vi "channel.data_type.vi"(8 "error in":errorcluster, 11 "Channel in":refnum<class "Channel.lvclass">) -> (0 "error out":errorcluster, 2 "type":i32, 3 "Channel out":refnum<class "Channel.lvclass">)   [LabVIEW 2020, in "Channel.lvclass"]
doc: "Returns the channel's data type."
uses:
  Channel.lvclass
  Channel.lvclass/Channel.ctl
  client.lvlib
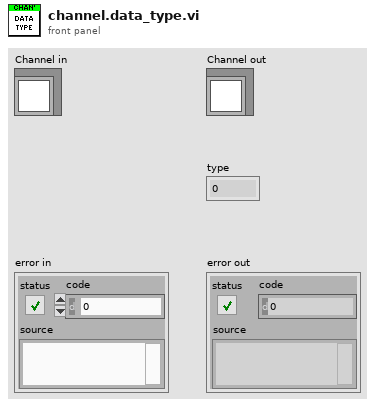
[diagram p1: front panel]
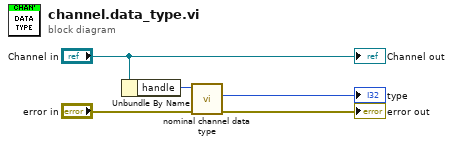
[diagram p0: block diagram]
diagram:
  n1 = Unbundle By Name("Channel in") -> ("handle"=w3:i32)
  n2 = call "nominal channel data type.vi"("error in (no error)"="error in", "channel"=w3) -> ("error out"=→"error out":errorcluster, "out_type out"=→"type":i32)  [unwired: 7 in, 1 out]
  "Channel out" <- "Channel in"
